vi "Actor Core.vi"(8 "error in":errorcluster, 11 "HIJ JETI100 F and E Camera In":refnum<class "HIJ Vision App Fluence and Energy Camera.lvclass">) -> (0 "error out":errorcluster, 3 "Actor out":refnum<class "Actor.lvclass">)   [LabVIEW 2014, in "HIJ Vision App Fluence and Energy Camera.lvlib" / "HIJ Vision App Fluence and Energy Camera.lvclass"]
doc: "(<B>Filename</B>: Actor Framework.lvlib:Actor.lvclass:Actor Core.vi)\n\nReceives messages to the actor, reacts to them, and initiates any error handling that may shut the actor down.\n\nDescendant classes may override this VI to append parallel tasks for the actor to complete while it handles messages. Overrides use the Call Parent Method node."
uses:
  HIJ Vision App Fluence and Energy Camera.lvclass
  <vilib>/ActorFramework/Actor/Actor.lvclass
  Display Actors/HIJ IMAQdx Display/AF IMAQ Display/HIJ IMAQdx Display.lvclass
  Analyze/Analyze Classes/Analyze Diviation/Analyze BeamDeviation.lvclass
  Analyze/Results and Overlays/Results Beam Deviation/Analyze Results Beam Deviation.lvclass
  Camera Actors/IMAQdx Actor/IMAQdx Actor/IMAQdx Actor.lvclass
  Analyze/Results and Overlays/Results Fluence/Analyze Results Fluence.lvclass
  Analyze/Analyze Parameter/Analyze Parameter Fluence/Analyze Parameter Fluence.lvclass
  Analyze/Analyze Classes/Analyze Fluence and Energy/Analyze Fluence and Energy.lvclass
  Analyze/Results and Overlays/Results Energy/Analyze Results Energy.lvclass
  Analyze/Analyze Parameter/Analyze Parameter Energy per Count/Analyze Parameter Energy per Count.lvclass
  Display Actors/HIJ Vision Display/HIJ Vision Display/HIJ Vision Display.lvclass/HIJ Vision Display.ctl
  HIJ Vision App Fluence and Energy Camera.lvclass/HIJ Vision App Fluence and Energy Camera.ctl
  Analyze/Analyze Parameter/Analyze Parameter Energy per Count/Analyze Parameter Energy per Count.lvclass/Analyze Parameter Energy per Count.ctl
  Analyze/Results and Overlays/Results Fluence/Analyze Results Fluence.lvclass/Analyze Results Fluence.ctl
  Analyze/Results and Overlays/Results Energy/Analyze Results Energy.lvclass/Analyze Results Energy.ctl
  HIJ Vision Application/HIJ Vision Application/HIJ Vision Application.lvclass/HIJ Vision Application.ctl
  HIJ Vision Camera App/HIJ Vision Camera App/HIJ Vision Camera App.lvclass/HIJ Vision Camera App.ctl
  Shared Code/Viewable Actor/ViewableActor/ViewableActor.lvclass/ViewableActor.ctl
  <vilib>/ActorFramework/Actor/Actor.lvclass/Actor.ctl
  <vilib>/ActorFramework/Message Enqueuer/Message Enqueuer.lvclass/Message Enqueuer.ctl
  HIJ Vision Camera App/HIJ Vision Camera App Messages/Menu Selection Msg/Menu Selection Msg.lvclass/Menu Selection Msg.ctl
  Display Actors/HIJ Vision Display/HIJ Vision Display/Write Save Report_.vi
  Analyze/Results and Overlays/Results Fluence/Write UI Ref Max F.vi
  Analyze/Results and Overlays/Results Energy/Write UI Ref.vi
  Analyze/Analyze Parameter/Analyze Parameter Energy per Count/Write J_count.vi
  HIJ Vision Application/HIJ Vision Application/Write SubPnl for Display.vi
  HIJ Vision Camera App/HIJ Vision Camera App/Write Child Menu.vi
  HIJ Vision Application/HIJ Vision Application/Write HIJ Vision Display.vi
  HIJ Vision Camera App/HIJ Vision Camera App/Write Camera Actor.vi
  Shared Code/Viewable Actor/ViewableActor/Write UI VI Ref.vi
  HIJ Vision Application/HIJ Vision Application/Write Analyze Objs.vi
  <vilib>/ActorFramework/Message Enqueuer/Init from Existing Queue.vi
  <vilib>/ActorFramework/Message Enqueuer/Enqueue.vi
  <vilib>/ActorFramework/Message Priority Queue/Priority Enqueue.vi
  <vilib>/ActorFramework/Message Enqueuer/Message Enqueuer.lvclass
  HIJ Vision Camera App/HIJ Vision Camera App Messages/Menu Selection Msg/Menu Selection Msg.lvclass
  <vilib>/ActorFramework/Stop Msg/Stop Msg.lvclass
  HIJ Vision Camera App/HIJ Vision Camera App/HIJ Vision Camera App.lvclass
panel:
  in  "Stop Button":bool
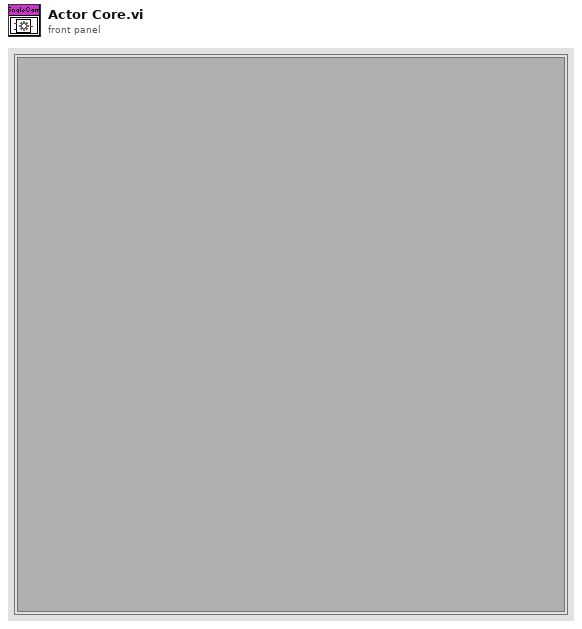
[diagram p1: front panel]
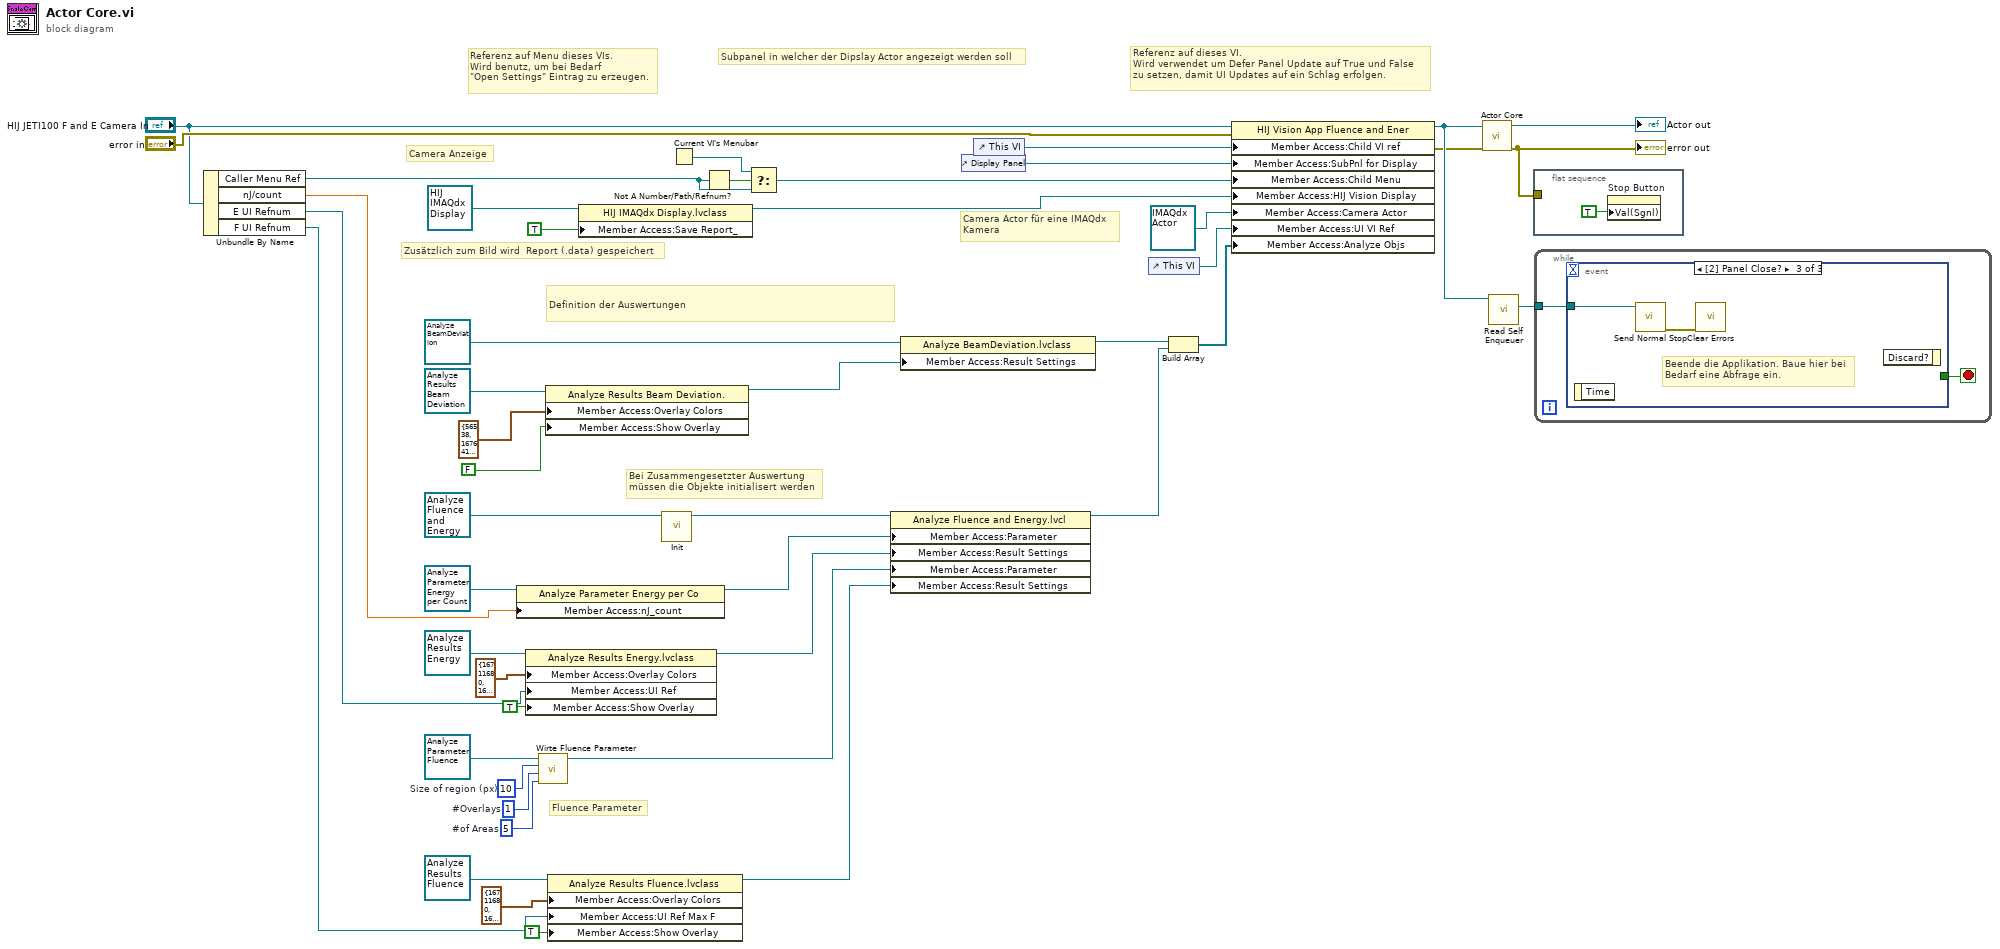
[diagram p0: block diagram]
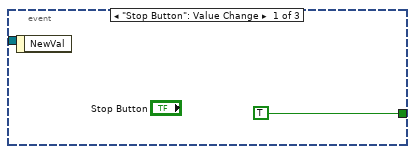
[diagram p2: hidden frame]
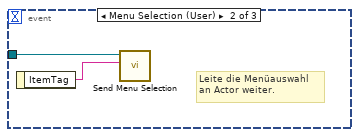
[diagram p3: hidden frame]
diagram:
  w24 = 10  # Size of region (px)
  w25 = 1  # #Overlays
  w26 = 5  # #of Areas
  # "Bei Zusammengesetzter Auswertung \nmüssen die Objekte initialisert werden"
  # "Camera Actor für eine IMAQdx\nKamera"
  # "Referenz auf Menu dieses VIs.\nWird benutz, um bei Bedarf \n\"Open Settings\" Eintrag zu erzeugen."
  # "Fluence Parameter"
  # "Referenz auf dieses VI.\nWird verwendet um Defer Panel Update auf True und False\nzu setzen, damit UI Updates auf ein Schlag erfolgen."
  # "Definition der Auswertungen"
  # "Camera Anzeige"
  # "Zusätzlich zum Bild wird  Report (.data) gespeichert"
  # "Subpanel in welcher der Dipslay Actor angezeigt werden soll"
  n1 = Unbundle By Name("HIJ JETI100 F and E Camera In") -> ("Caller Menu Ref"=w18:refnum<k9>, "nJ/count"=w12:dbl[unit], "E UI Refnum"=w4:refnum<vi>, "F UI Refnum"=w3:refnum<vi>)
  n2 = property class="Analyze Parameter Energy per Co"(reference=refnum<class "Analyze Parameter Energy per Count.lvclass"> refnum ("Analyze Parameter Energy per Count.lvclass"), "Member Access:nJ_count"=w12) -> (reference out=w8:refnum<class "Analyze Parameter Energy per Count.lvclass">)  [unwired: 1 in, 1 out]
  n3 = property class="Analyze Results Energy.lvclass"(reference=refnum<class "Analyze Results Energy.lvclass"> refnum ("Analyze Results Energy Obj"), "Member Access:Overlay Colors"=cluster{"Border":u32, "Text":u32} {"Border"=16711680, "Text"=16448250} ("Colors"), "Member Access:UI Ref"=w4, "Member Access:Show Overlay"=TRUE ("Show Overlay")) -> (reference out=w7:refnum<class "Analyze Results Energy.lvclass">)  [unwired: 1 in, 1 out]
  n4 = call "Wirte Fluence Parameter.vi"("#of Areas"=w26, "#Overlays"=w25, "Size of region (px)"=w24, "Analyze Parameter Fluence in"=refnum<class "Analyze Parameter Fluence.lvclass"> refnum ("Analyze Parameter Fluence.lvclass")) -> ("Analyze Parameter Fluence out"=w6:refnum<class "Analyze Parameter Fluence.lvclass">)  [unwired: 7 in]
  n5 = property class="Analyze Results Beam Deviation."(reference=refnum<class "Analyze Results Beam Deviation.lvclass"> refnum ("Analyze Results Beam Deviation.lvclass"), "Member Access:Overlay Colors"=cluster{"Border":u32, "Text":u32} {"Border"=56538, "Text"=16764160} ("Colors"), "Member Access:Show Overlay"=FALSE ("Show Overlay")) -> (reference out=w28:refnum<class "Analyze Results Beam Deviation.lvclass">)  [unwired: 1 in, 1 out]
  n6 = property class="Analyze Results Fluence.lvclass"(reference=refnum<class "Analyze Results Fluence.lvclass"> refnum ("Analyze Results Fluence.lvclass"), "Member Access:Overlay Colors"=cluster{"Border":u32, "Text":u32} {"Border"=16711680, "Text"=16448250} ("Colors"), "Member Access:UI Ref Max F"=w3, "Member Access:Show Overlay"=TRUE ("Show Overlay")) -> (reference out=w5:refnum<class "Analyze Results Fluence.lvclass">)  [unwired: 1 in, 1 out]
  n7 = property class="HIJ IMAQdx Display.lvclass"(reference=refnum<class "HIJ IMAQdx Display.lvclass"> refnum ("IMAQ Display.lvlib:IMAQ Display.lvclass"), "Member Access:Save Report_"=TRUE ("Save Report_")) -> (reference out=w31:refnum<class "HIJ IMAQdx Display.lvclass">)  [unwired: 1 in, 1 out]
  n8 = call "Init.vi"("Analyze Fluence and Energy in"=refnum<class "Analyze Fluence and Energy.lvclass"> refnum ("Analyze.lvlib:Analyze Fluence and Energy.lvclass")) -> ("Analyze Fluence and Energy out"=w10:refnum<class "Analyze Fluence and Energy.lvclass">)  [unwired: 9 in, 1 out]
  n9 = Current VI's Menubar() -> (w19:refnum<k9>)
  n10 = Not A Number/Path/Refnum?(number/path/refnum=w18) -> (NaN/Path/Refnum?=w21:bool)
  n11 = Select(t=w19, s=w21, f=w18) -> (s? t:f=w20:refnum<k9>)
  n12 = property class="Analyze Fluence and Energy.lvcl"(reference=w10, "Member Access:Parameter"=w8, "Member Access:Result Settings"=w7, "Member Access:Parameter"=w6, "Member Access:Result Settings"=w5) -> (reference out=w9:refnum<class "Analyze Fluence and Energy.lvclass">)  [unwired: 1 in, 1 out]
  n13 = property class="Analyze BeamDeviation.lvclass"(reference=refnum<class "Analyze BeamDeviation.lvclass"> refnum ("Analyze.lvlib:Analyze BeamDeviation.lvclass"), "Member Access:Result Settings"=w28) -> (reference out=w29:refnum<class "Analyze BeamDeviation.lvclass">)  [unwired: 1 in, 1 out]
  n14 = control-ref of="Display Panel"() -> (w33:refnum<vi>)
  n15 = control-ref of="This VI"() -> (w36:refnum<vi>)
  n16 = control-ref of="This VI"() -> (w23:refnum<vi>)
  n17 = Build Array(w29, w9) -> (w15:refnum<class "Analyze BaseClass.lvclass">[])
  n18 = property class="HIJ Vision App Fluence and Ener"(reference="HIJ JETI100 F and E Camera In", error in="error in", "Member Access:Child VI ref"=w36, "Member Access:SubPnl for Display"=w33, "Member Access:Child Menu"=w20, "Member Access:HIJ Vision Display"=w31, "Member Access:Camera Actor"=refnum<class "IMAQdx Actor.lvclass"> refnum ("IMAQdx Actor.lvlib:IMAQdx Actor.lvclass"), "Member Access:UI VI Ref"=w23, "Member Access:Analyze Objs"=w15) -> (reference out=w37:refnum<class "HIJ Vision App Fluence and Energy Camera.lvclass">, error out=w34:errorcluster)
  n19 = call-parent "Actor Core.vi"("error in"=w34, "HIJ Vision Camera App In"=w37) -> ("error out"=w43:errorcluster, "Actor out"=→"Actor out":refnum<class "Actor.lvclass">)  [unwired: 8 in]
  "error out" <- w43
  n20 = call <vilib>:"Read Self Enqueuer.vi"("Actor"=w37) -> ("Self Enqueuer"=w42:refnum<class "Message Enqueuer.lvclass">)  [unwired: 10 in]
  n21 = flat-sequence {
    tunnel: w43 -> [_]
    frame #0 {
      n22 = property on="Stop Button" class="Bool (strict)"("Val(Sgnl)"=TRUE) -> ()  [unwired: 2 in, 2 out]
    }
  }
  n23 = while {
    tunnel: w42 -> [w48]
    stop <- w49 stop-if-true
    n24 = event shown="[2] Panel Close?" {
      selector: _ -> [_ _ _]
      dyn-events: _ -> [_ _ _]
      timeout: _ -> [_ _ _]
      tunnel: [TRUE _ _] -> w49
      tunnel: w48 -> [_ w51 w54]
      event "Stop Button": Value Change {
        n25 = event-data() -> ()  [unwired: 1 in, 1 out]
      }
      event Menu Selection (User) {
        # "Leite die Menüauswahl \nan Actor weiter."
        n26 = event-data() -> ("ItemTag"=w52:string)  [unwired: 1 in]
        n27 = call "Send Menu Selection.vi"("MenuTag"=w52, "Message Enqueuer"=w51) -> ()  [unwired: 8 in, 2 out]
      }
      event Panel Close? {
        # "Beende die Applikation. Baue hier bei\nBedarf eine Abfrage ein."
        n28 = event-data() -> ()  [unwired: 1 in, 1 out]
        n29 = call <vilib>:"Send Normal Stop.vi"("Message Enqueuer"=w54) -> ("error out"=w53:errorcluster)  [unwired: 10 in]
        n30 = call <vilib>:"Clear Errors.vi"("error in (no error)"=w53) -> ()  [unwired: 5 in, 2 out]
        n31 = event-data() -> ()  [unwired: 2 in, 1 out]
      }
    }
  }
